vi "Attack.vi"(8 "error in (no error)":errorcluster, 11 "Test in":refnum<class "Swarm.lvclass">) -> (0 "error out":errorcluster, 3 "Test out":refnum<class "Swarm.lvclass">)   [LabVIEW 2017, in "Swarm.lvclass"]
uses:
  Swarm.lvclass
  Swarm.lvclass/Swarm.ctl
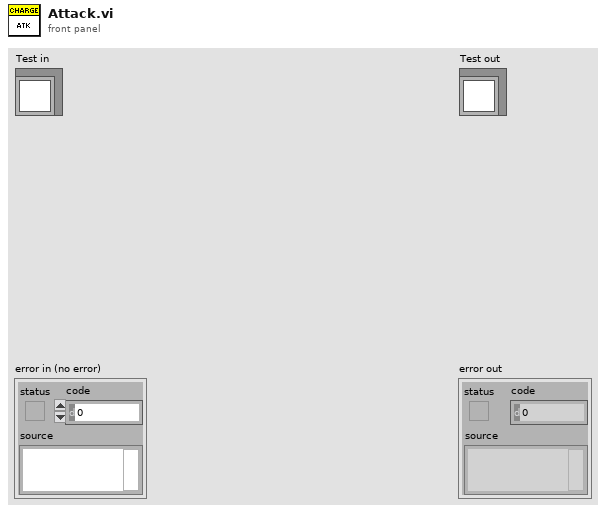
[diagram p1: front panel]
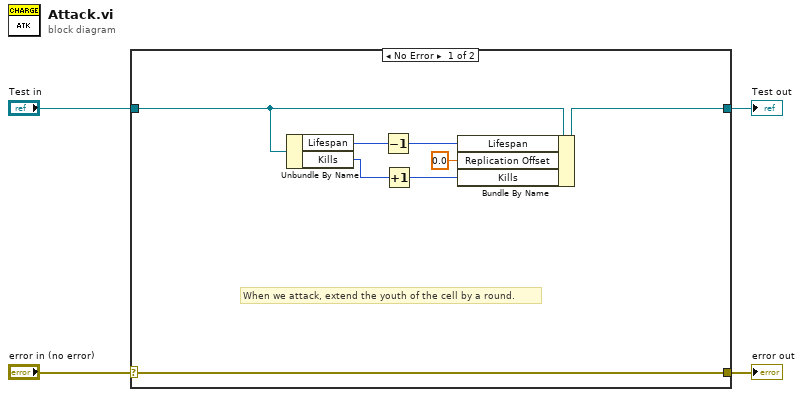
[diagram p0: block diagram]
diagram:
  n1 = case shown="No Error" "error in (no error)" {
    selector: "error in (no error)" -> [w12 w14]
    tunnel: [w12 w14] -> w3
    tunnel: [w8 w13] -> w1
    tunnel: "Test in" -> [w9 w13]
    frame No Error {
      # "When we attack, extend the youth of the cell by a round."
      n2 = Unbundle By Name(w9) -> ("Lifespan"=w11:i32, "Kills"=w6:i32)
      n3 = Decrement(x=w11) -> (x-1=w10:i32)
      n4 = Increment(x=w6) -> (x+1=w5:i32)
      n5 = Bundle By Name(cluster=w9, "Lifespan"=w10, "Replication Offset"=0.0, "Kills"=w5) -> (w8:refnum<class "Swarm.lvclass">)
    }
    frame Error {
    }
  }
  "error out" <- w3
  "Test out" <- w1
